vi "Panchita.vi"() -> ()   [LabVIEW 2017]
panel:
  in  "Para":bool
  out "Guia":bool
  out "Glo":bool
  out "Que":bool
  out "Sol":bool
  out "Info":bool
  in  "Glo":bool
  in  "Info":bool
  in  "Guia":bool
  in  "Queja":bool
  in  "Solicitud":bool
  in  "Panchita 2":bool caption="Panchita"
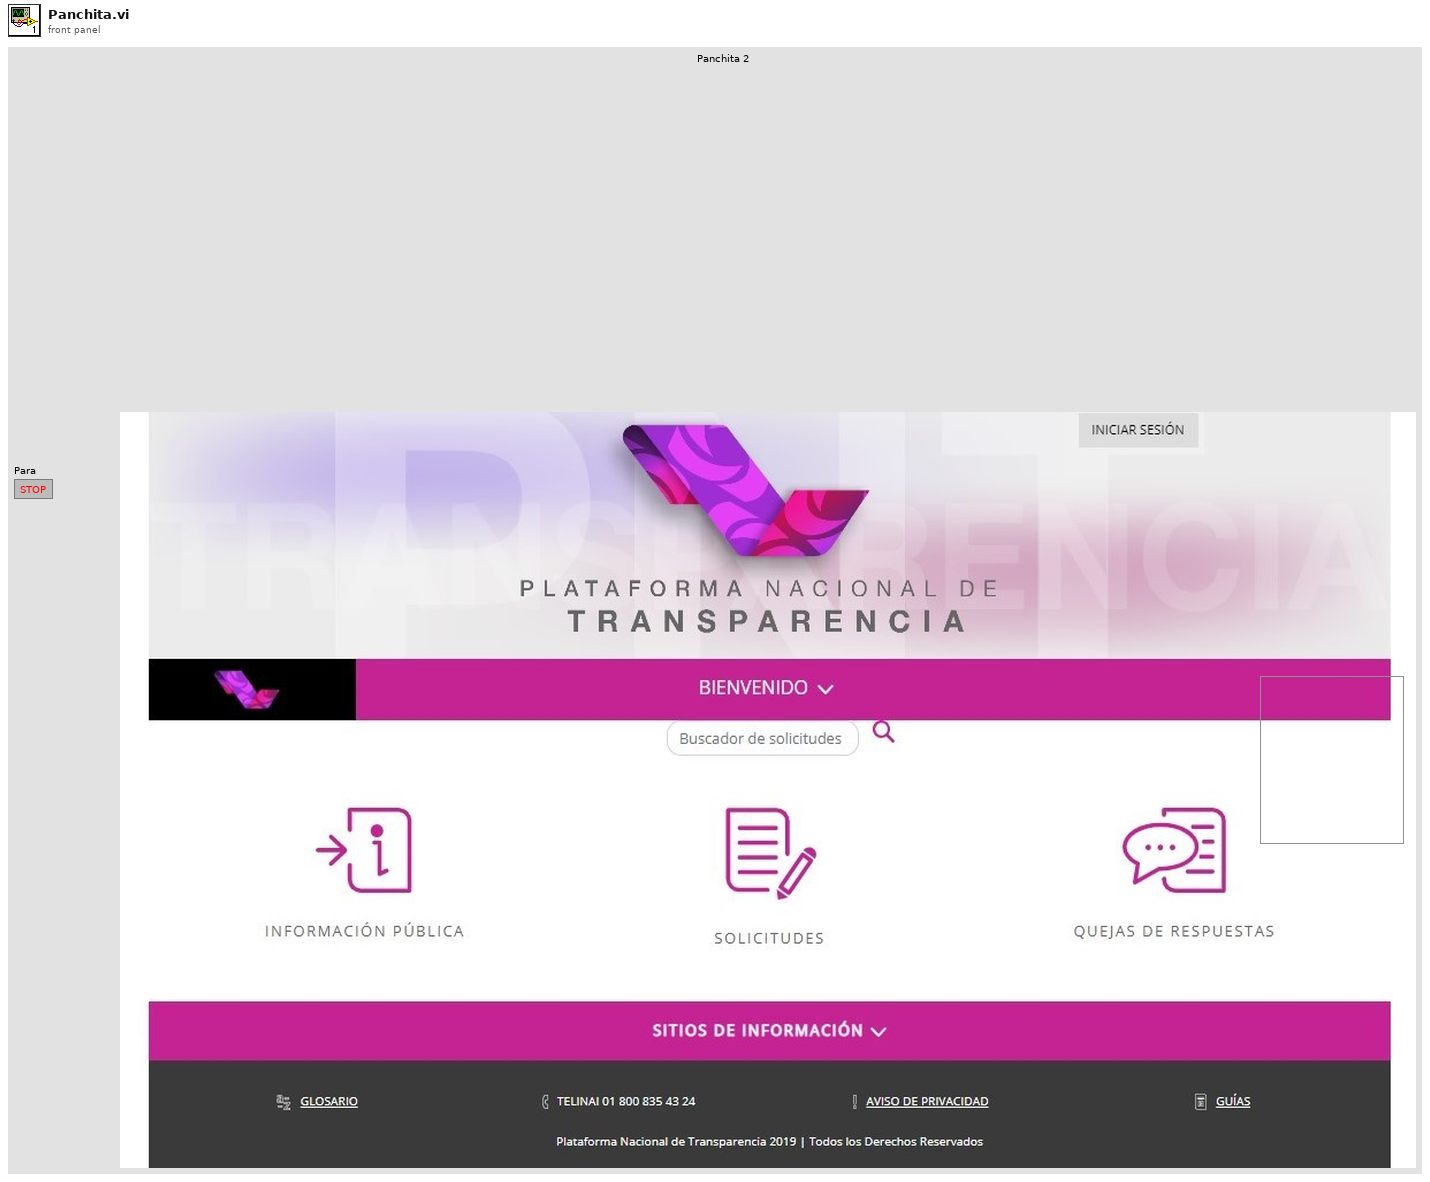
[diagram p1: front panel]
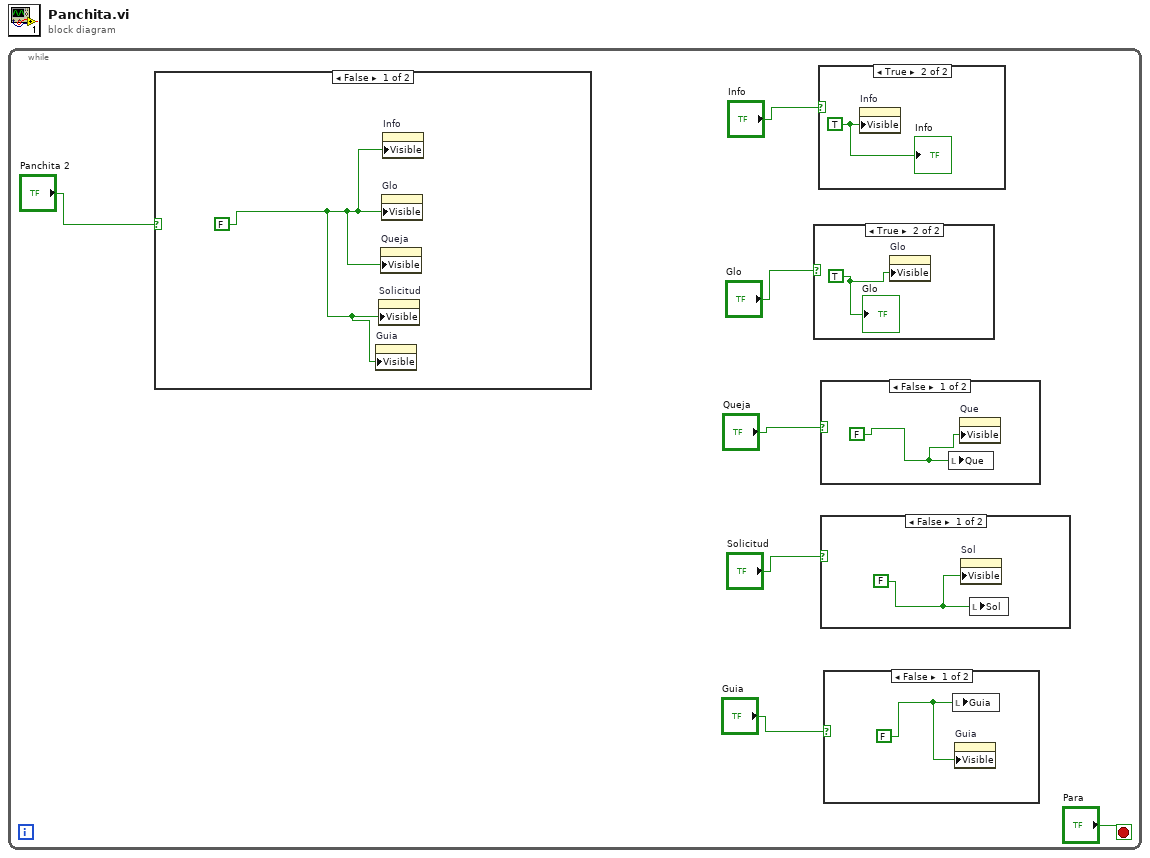
[diagram p0: block diagram]
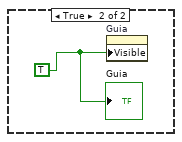
[diagram p2: hidden frame]
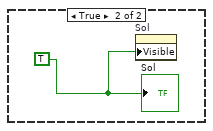
[diagram p3: hidden frame]
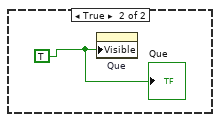
[diagram p4: hidden frame]
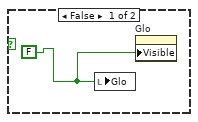
[diagram p5: hidden frame]
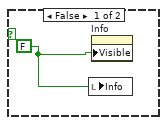
[diagram p6: hidden frame]
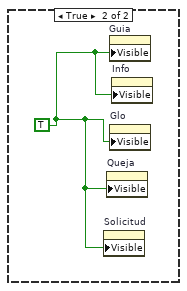
[diagram p7: hidden frame]
diagram:
  n1 = while {
    stop <- "Para" stop-if-true
    n2 = case shown="False" "Panchita 2" {
      frame False {
        w18 = FALSE
        n3 = property on="Guia" class="Bool (strict)"("Visible"=w18) -> ()  [unwired: 2 in, 2 out]
        n4 = property on="Solicitud" class="Bool (strict)"("Visible"=w18) -> ()  [unwired: 2 in, 2 out]
        n5 = property on="Queja" class="Bool (strict)"("Visible"=w18) -> ()  [unwired: 2 in, 2 out]
        n6 = property on="Glo" class="Bool (strict)"("Visible"=w18) -> ()  [unwired: 2 in, 2 out]
        n7 = property on="Info" class="Bool (strict)"("Visible"=w18) -> ()  [unwired: 2 in, 2 out]
      }
      frame True {
        w19 = TRUE
        n8 = property on="Solicitud" class="Bool (strict)"("Visible"=w19) -> ()  [unwired: 2 in, 2 out]
        n9 = property on="Queja" class="Bool (strict)"("Visible"=w19) -> ()  [unwired: 2 in, 2 out]
        n10 = property on="Guia" class="Bool (strict)"("Visible"=w19) -> ()  [unwired: 2 in, 2 out]
        n11 = property on="Glo" class="Bool (strict)"("Visible"=w19) -> ()  [unwired: 2 in, 2 out]
        n12 = property on="Info" class="Bool (strict)"("Visible"=w19) -> ()  [unwired: 2 in, 2 out]
      }
    }
    n13 = case shown="True" "Glo" {
      frame False {
        w14 = FALSE
        n14 = local write "Glo"(w14) -> ()
        n15 = property on="Glo" class="Bool (strict)"("Visible"=w14) -> ()  [unwired: 2 in, 2 out]
      }
      frame True {
        w15 = TRUE
        n16 = property on="Glo" class="Bool (strict)"("Visible"=w15) -> ()  [unwired: 2 in, 2 out]
        "Glo" <- w15
      }
    }
    n17 = case shown="True" "Info" {
      frame False {
        w16 = FALSE
        n18 = local write "Info"(w16) -> ()
        n19 = property on="Info" class="Bool (strict)"("Visible"=w16) -> ()  [unwired: 2 in, 2 out]
      }
      frame True {
        w17 = TRUE
        n20 = property on="Info" class="Bool (strict)"("Visible"=w17) -> ()  [unwired: 2 in, 2 out]
        "Info" <- w17
      }
    }
    n21 = case shown="False" "Queja" {
      frame False {
        w12 = FALSE
        n22 = local write "Que"(w12) -> ()
        n23 = property on="Que" class="Bool (strict)"("Visible"=w12) -> ()  [unwired: 2 in, 2 out]
      }
      frame True {
        w13 = TRUE
        n24 = property on="Que" class="Bool (strict)"("Visible"=w13) -> ()  [unwired: 2 in, 2 out]
        "Que" <- w13
      }
    }
    n25 = case shown="False" "Solicitud" {
      frame False {
        w10 = FALSE
        n26 = property on="Sol" class="Bool (strict)"("Visible"=w10) -> ()  [unwired: 2 in, 2 out]
        n27 = local write "Sol"(w10) -> ()
      }
      frame True {
        w11 = TRUE
        n28 = property on="Sol" class="Bool (strict)"("Visible"=w11) -> ()  [unwired: 2 in, 2 out]
        "Sol" <- w11
      }
    }
    n29 = case shown="False" "Guia" {
      frame False {
        w8 = FALSE
        n30 = local write "Guia"(w8) -> ()
        n31 = property on="Guia" class="Bool (strict)"("Visible"=w8) -> ()  [unwired: 2 in, 2 out]
      }
      frame True {
        w9 = TRUE
        n32 = property on="Guia" class="Bool (strict)"("Visible"=w9) -> ()  [unwired: 2 in, 2 out]
        "Guia" <- w9
      }
    }
  }
